vi "Compute Controller Ouput.vi"(4 "Phase":dbl, 6 "HS":bool, 8 "Setpoint":dbl, 11 "State":T1) -> (0 "Full Output":dbl)   [LabVIEW 2018]
uses:
  State.ctl
  Feedback Control/Feedback Controller Gains.ctl
  Feedback Control/COBRA Feedback Control Library.lvlib
  COBRA Iterative Learning Control Library.lvlib
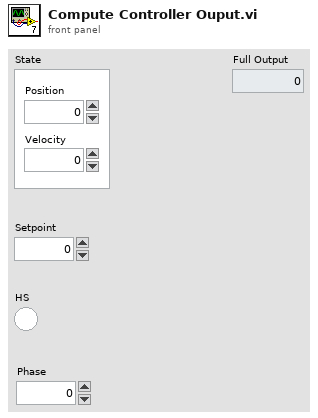
[diagram p1: front panel]
types:
  T1 = typedef "State.ctl" = cluster{"Position":dbl, "Velocity":dbl}
  T2 = typedef "COBRA Feedback Control Library.lvlib/Feedback Controller Gains.ctl" = cluster{"Kp":dbl, "Kd":dbl}
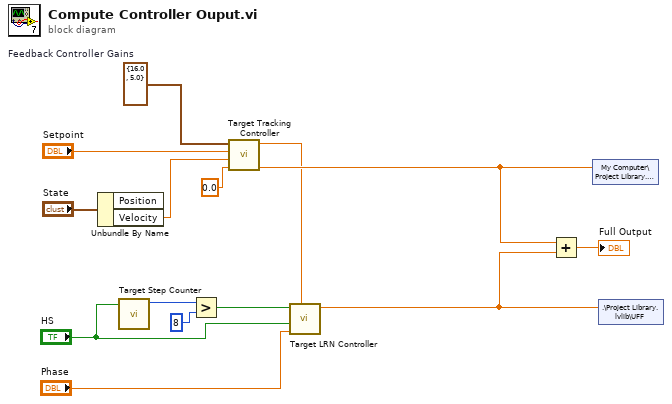
[diagram p0: block diagram]
diagram:
  w14 = T2 {"Kp"=16.0, "Kd"=5.0}  # Feedback Controller Gains
  n1 = Unbundle By Name("State") -> ("Velocity"=w7:dbl)  [unwired: 1 out]
  n2 = call "Target Step Counter.vi"("HS"="HS") -> ("Number of Steps"=w10:i64)  [unwired: 10 in]
  n3 = Greater?(x=w10, y=i64 8) -> (0:w5:bool)
  n4 = call "Target Tracking Controller.vi"("Motor Velocity (deg/s)"=0.0, "Filtered Force (N)"=w7, "Force Setpoint (N)"="Setpoint", "Feedback Controller Gains"=w14) -> ("Motor Velocity Command (deg/s)"=w6:dbl, "Error (N)"=w4:dbl)  [unwired: 6 in]
  n5 = call "Target LRN Controller.vi"("Error"=w4, "Phase"="Phase", "HS"="HS", "Active?"=w5) -> ("UFF"=w1:dbl)  [unwired: 7 in]
  n6 = Add(x=w6, y=w1) -> (x+y=→"Full Output":dbl)
  n7 = shared-variable "My Computer\\Project Library.lvlib\\UFB"(w6) -> ()  [unwired: 1 in, 1 out]
  n8 = shared-variable ".\\Project Library.lvlib\\UFF"(w1) -> ()  [unwired: 1 in, 1 out]
